vi "De-queue RT schedule element.vi"(11 "RT Queues":T2) -> (1 "scheduled message":T1, 3 "Action":enum16{"New", "Remove", "Quit"}(ring), 4 "timeout":bool)   [LabVIEW 2018]
uses:
  Type Defs/scheduled message cluster.ctl
  Message Scheduler/Message scheduler.lvlib
  Type Defs/Queues cluster.ctl
  Queues.lvlib
  Chris VIs/Message Scheduler/message scheduler.lvclass
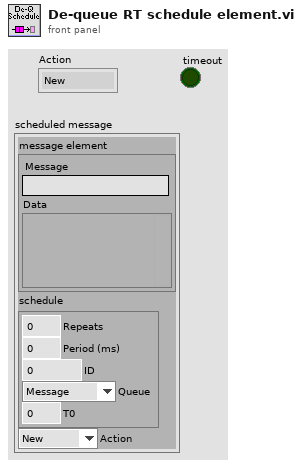
[diagram p1: front panel]
types:
  T1 = typedef "Real-Time.lvlib/Message scheduler.lvlib/scheduled message cluster.ctl" = cluster{"message element":cluster{"Message":string, "Data":variant}, "schedule":cluster{"Repeats":i16, "Period (ms)":u32, "ID":u32, "Queue":enum16{"Message", "Comms"}, "T0":u32}, "Action":enum16{"New", "Remove", "Quit"}}
  T2 = typedef "Real-Time.lvlib/Queues.lvlib/Queues cluster.ctl" = cluster{"RT Message":refnum<queue>, "RT Comms":refnum<queue>, "RT Data":refnum<queue>, "message scheduler":refnum<class "message scheduler.lvclass">}
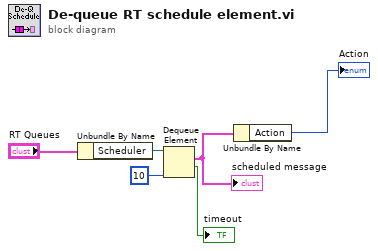
[diagram p0: block diagram]
diagram:
  n1 = Unbundle By Name("RT Queues") -> ("Scheduler"=w5:refnum<queue>)
  n2 = Dequeue Element(queue=w5, timeout in ms (-1)=10) -> (element=w4:T1, timed out?=→"timeout":bool)  [unwired: 1 in, 2 out]
  "scheduled message" <- w4
  n3 = Unbundle By Name(w4) -> ("Action"=→"Action":enum16{"New", "Remove", "Quit"})
